vi "RT Main.vi"() -> ()   [LabVIEW 2014]
doc: "This example is based on the MAX5216. It allows you to control the voltage output on the SPI chip. This VI interfaces with the SPI Engine on the FPGA."
uses:
  <vilib>/FPGAPlugInAG/sbRIO-9651/niLvFpga_Open_sbRIO-9651.vi
  <vilib>/rvi/interface/common/dynamic/niFpgaDynamicAddResources.vi
  <vilib>/FPGAPlugInAG/Dynamic/niLvFpga_Reset_Dynamic.vi
  <vilib>/FPGAPlugInAG/Dynamic/niLvFpga_Run_Dynamic.vi
  <vilib>/Utility/error.llb/Error Cluster From Error Code.vi
  <vilib>/rvi/errors/niLvFpgaAdjustHostInterfaceError.vi
  <vilib>/FPGAPlugInAG/Dynamic/niLvFpga_Close_Dynamic.vi
  <vilib>/rvi/interface/nirviOpenFPGA/nirviOpenFPGA.xnode
  FPGA Bitfiles/SPI Simple DAC Example.lvbitx
  <vilib>/rvi/interface/nirviMethod/nirviMethod.xnode
  <vilib>/rvi/interface/nirviReadWriteControl/nirviReadWriteControl.xnode
  <vilib>/rvi/interface/nirviCloseFPGA/nirviCloseFPGA.xnode
  <vilib>/rvi/interface/Simulation/niFpgaSimulationCallBeginRW.vi
  NiFpgaLv.dll
panel:
  in  "Reference Voltage":dbl=3.0 format="%f"
  out "Binary to DAC":u64 format="%024b"
  in  "Voltage Output":dbl=3.0 format="%f"
  in  "data rate (S/s)":u32=10
  in  "SPI PHY Settings":T1={"Divide Value"=20, "Transfer Length (bits)"=24, "CS Asserted Polarity"=FALSE, "Clock Polarity (CPOL)"=FALSE, "Clock Phase (CPHA)"=FALSE, "Lengthen MISO Setup"=FALSE, "Direction Change Bit"=0, "MOSI Starts as Output"=FALSE, "Tristatable MOSI"=FALSE}
  in  "stop":bool
  # "SPI Settings"
  # "Overview: This example is based on the MAX5216.  It allows you to control the\nvoltage output on the SPI chip. \nRequirements: LabVIEW Full Development System, LabVIEW Real Time, \nLabVIEW FPGA, MAX5216, NI System on Module, NI 9651.\nInstructions:\n1. The SPI PHY Settings are already setup for the MAX5216.  Do not adjust them.\n2. Plug the MAX5216 into PMOD1 on the NI 9651.\n3. Setup Vref according to the user manual.\n4. Run the VI.\n5. Adjust the Voltage Output and observe the voltage change on the MAX5216."
  # "MSB"
  # "LSB"
  # "Sampling Info"
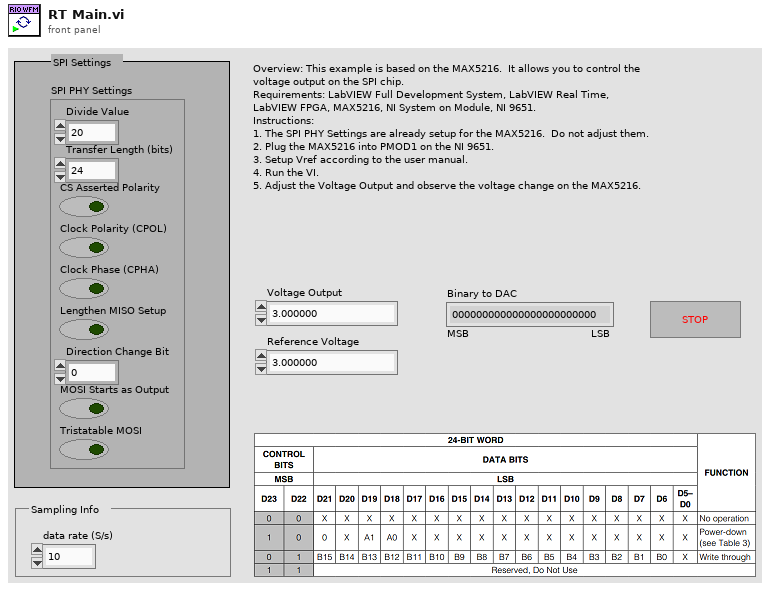
[diagram p1: front panel]
types:
  T1 = cluster{"Divide Value":u8, "Transfer Length (bits)":u8, "CS Asserted Polarity":bool, "Clock Polarity (CPOL)":bool, "Clock Phase (CPHA)":bool, "Lengthen MISO Setup":bool, "Direction Change Bit":u8, "MOSI Starts as Output":bool, "Tristatable MOSI":bool}
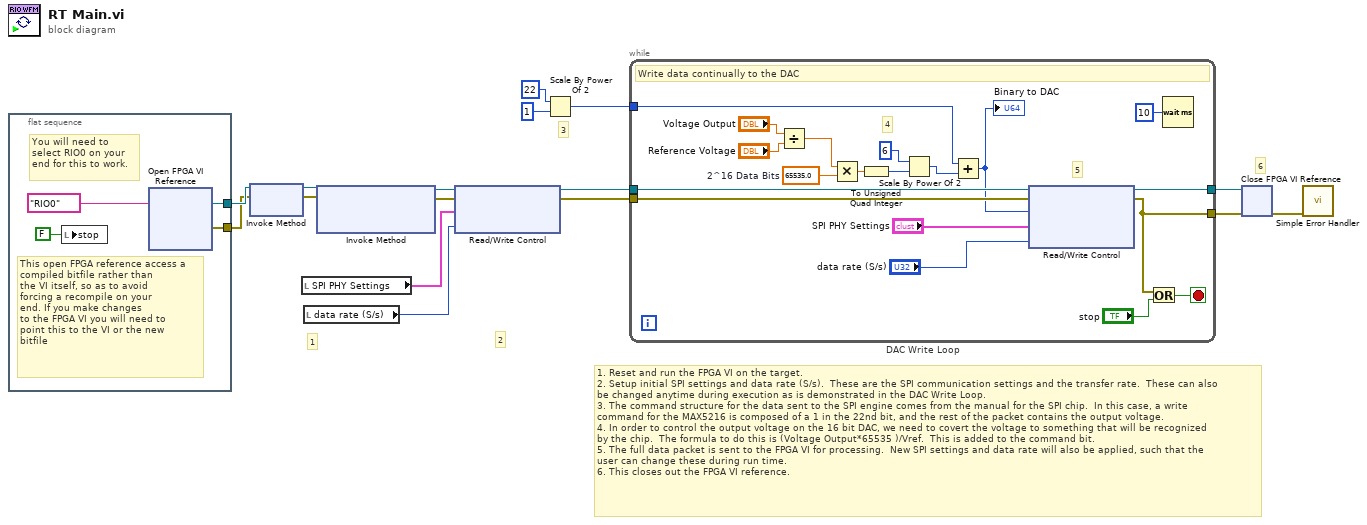
[diagram p0: block diagram]
diagram:
  # "1. Reset and run the FPGA VI on the target.\n2. Setup initial SPI settings and data rate (S/s).  These are the SPI communication settings and the transfer rate.  These can also\nbe changed anytime during execution as is demonstrated in the DAC Write Loop.\n3. The command structure for the data sent to the SPI engine comes from the manual for the SPI chip.  In this case, a write\ncommand for the MAX5216 is composed of a 1 in the 22nd bit, and the rest of the packet contains the output voltage.\n4. In order to control the output voltage on the 16 bit DAC, we need to covert the voltage to something that will be recognized\nby the chip.  The formula to do this is (Voltage Output*65535 )/Vref.  This is added to the command bit.\n5. The full data packet is sent to the FPGA VI for processing.  New SPI settings and data rate will also be applied, such that the\nuser can change these during run time.\n6. This closes out the FPGA VI reference."
  # "6"
  # "3"
  # "2"
  # "1"
  n1 = flat-sequence {
    tunnel: [w19] -> w16
    tunnel: [w18] -> w15
    frame #0 {
      # "You will need to\nselect RIO0 on your\nend for this to work."
      # "This open FPGA reference access a\ncompiled bitfile rather than \nthe VI itself, so as to avoid\nforcing a recompile on your\nend. If you make changes\nto the FPGA VI you will need to\npoint this to the VI or the new\nbitfile"
      n2 = local write "stop"(FALSE ("stop")) -> ()
      n3 = xnode "Open FPGA VI Reference"("resource name"=tag "RIO0") -> ("FPGA VI Reference Out"=w19:refnum<k20>, "error out"=w18:errorcluster)  [unwired: 1 in]
    }
  }
  n4 = xnode "Invoke Method"("FPGA VI Reference In"=w16, "error in"=w15) -> ("FPGA VI Reference Out"=w10:refnum<k20>, "error out"=w9:errorcluster)
  n5 = local read "SPI PHY Settings"() -> (w4:T1)
  n6 = local read "data rate (S/s)"() -> (w1:u32)
  n7 = xnode "Invoke Method"("FPGA VI Reference In"=w10, "error in"=w9) -> ("FPGA VI Reference Out"=w11:refnum<k20>, "error out"=w13:errorcluster)  [unwired: 1 in]
  n8 = xnode "Read/Write Control"("FPGA VI Reference In"=w11, "error in"=w13, "SPI PHY Settings"=w4, "data rate (S/s)"=w1) -> ("FPGA VI Reference Out"=w8:refnum<k20>, "error out"=w12:errorcluster)
  n9 = Scale By Power Of 2(n=i16 22, x=u64 1) -> (x*2^n=w5:u64)
  n10 = while "DAC Write Loop" {
    tunnel: w8 -> [w37]
    tunnel: w12 -> [w36]
    tunnel: w5 -> [w21]
    tunnel: [w34] -> w3
    tunnel: [w33] -> w2
    stop <- w39 stop-if-true
    w28 = 65535.0  # 2^16 Data Bits
    # "4"
    # "5"
    # "Write data continually to the DAC"
    n11 = Divide(x="Voltage Output", y="Reference Voltage") -> (x/y=w27:dbl)
    n12 = Multiply(x=w27, y=w28) -> (x*y=w26:dbl)
    n13 = To Unsigned Quad Integer(1:w26) -> (0:w25:u64)
    n14 = Scale By Power Of 2(n=i16 6, x=w25) -> (x*2^n=w23:u64)
    n15 = Add(x=w21, y=w23) -> (x+y=w22:u64)
    "Binary to DAC" <- w22
    n16 = xnode "Read/Write Control"("FPGA VI Reference In"=w37, "error in"=w36, "Data To DAC"=w22, "SPI PHY Settings"="SPI PHY Settings", "data rate (S/s)"="data rate (S/s)") -> ("FPGA VI Reference Out"=w34:refnum<k20>, "error out"=w33:errorcluster)
    n17 = Or(x=w33, y="stop") -> (x .or. y?=w39:bool)
    n18 = Wait (ms)(milliseconds to wait=u32 10) -> ()  [unwired: 1 out]
  }
  n19 = xnode "Close FPGA VI Reference"("FPGA VI Reference In"=w3, "error in"=w2) -> ("error out"=w14:errorcluster)
  n20 = call <vilib>:"Simple Error Handler.vi"("error in (no error)"=w14) -> ()  [unwired: 1 in, 8 out]
